vi "Read Data and Memory Array_RageATE.vi"(0 "VISA resource name":refnum<visa-resource-name>, 1 "Channel (1)":i32=1, 3 "Trace":i32=1, 5 "Source (0: Data)":u16(ring) items=["Data", "Memory"], 9 "Correction (0: Data)":u16(ring) items=["Formatted", "Corrected"], 11 "error in (no error)":errorcluster) -> (2 "dB":dbl[](array[numeric]), 4 "VISA resource name out":refnum<visa-resource-name>, 6 "Primary / Real":dbl[](array[numeric]), 10 "Secondary / Imaginary":dbl[](array[numeric]), 15 "error out":errorcluster)   [LabVIEW 2018, in "Agilent ENA Series.lvlib"]
doc: "Reads out the formated or corrected data or memory array, for the active trace of selected channel."
uses:
  Agilent ENA Series.lvlib
panel:
  out "size(s) 2":i32
  out "size(s)":i32
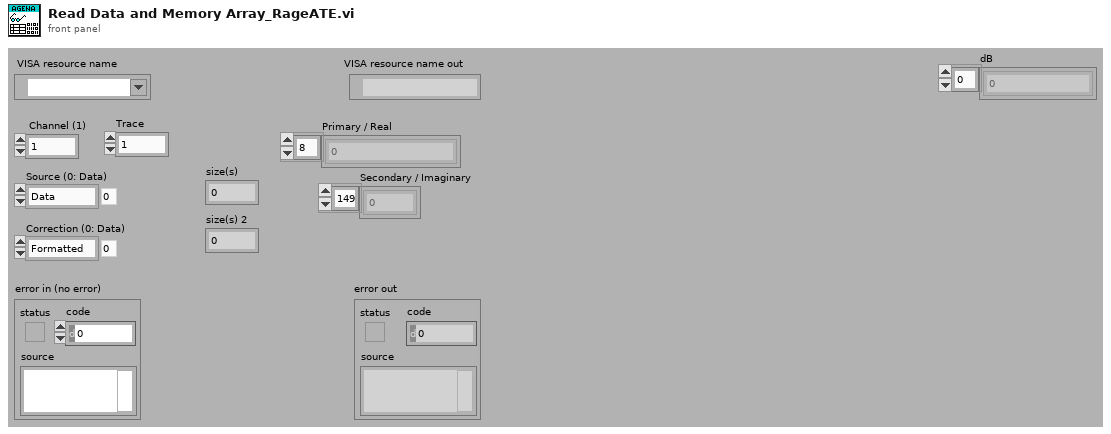
[diagram p1: front panel]
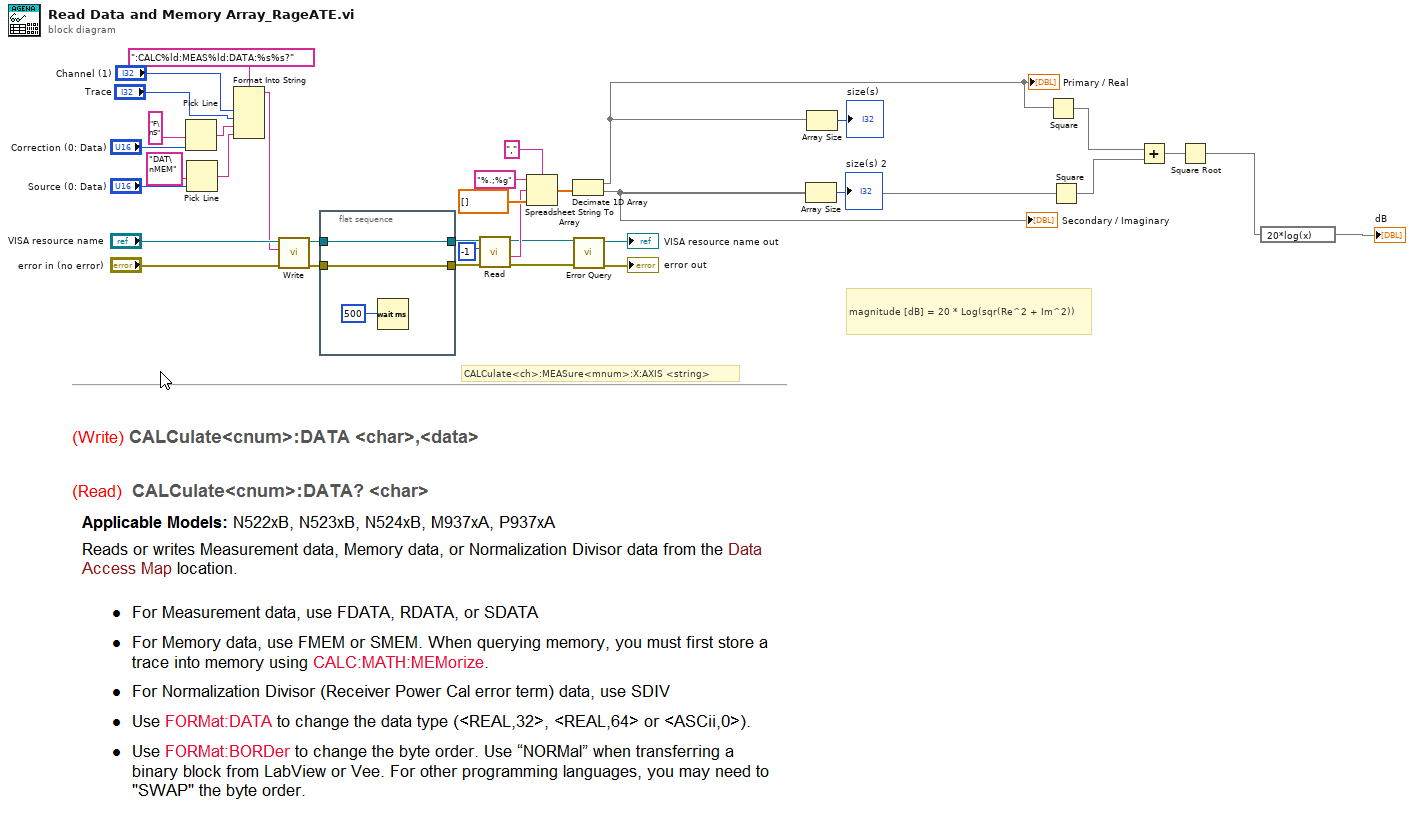
[diagram p0: block diagram]
diagram:
  # "magnitude [dB] = 20 * Log(sqr(Re^2 + Im^2))"
  # "CALCulate<ch>:MEASure<mnum>:X:AXIS <string>"
  n1 = Pick Line(multi-line string="F\nS", line index="Correction (0: Data)") -> (output string=w25:string)  [unwired: 1 in]
  n2 = Pick Line(multi-line string="DAT\nMEM", line index="Source (0: Data)") -> (output string=w22:string)  [unwired: 1 in]
  n3 = Format Into String(format string=":CALC%ld:MEAS%ld:DATA:%s%s?", "Channel (1)", "Trace", w25, w22) -> (resulting string=w31:string)  [unwired: 2 in, 1 out]
  n4 = call "Write.vi"("error in (no error)"="error in (no error)", "String ()"=w31, "VISA resource name"="VISA resource name") -> ("error out"=w16:errorcluster, "VISA resource name out"=w18:refnum<visa-resource-name>)  [unwired: 6 in, 1 out]
  n5 = flat-sequence {
    tunnel: w18 -> [w38]
    tunnel: [w38] -> w17
    tunnel: w16 -> [w37]
    tunnel: [w37] -> w15
    frame #0 {
      n6 = Wait (ms)(milliseconds to wait=u32 500) -> ()  [unwired: 1 out]
    }
  }
  n7 = call "Read.vi"("error in (no error)"=w15, "Number Of Bytes"=-1, "VISA resource name"=w17) -> ("error out"=w13:errorcluster, "String"=w21:string, "VISA resource name out"=w14:refnum<visa-resource-name>)  [unwired: 5 in, 1 out]
  n8 = Spreadsheet String To Array(delimiter (Tab)=",", format string="%.;%g", spreadsheet string=w21, array type (2D Dbl)=dbl[] []) -> (array=w19:dbl[])
  n9 = Decimate 1D Array(w19) -> (w7:dbl[], w6:dbl[])
  "Primary / Real" <- w7
  "Secondary / Imaginary" <- w6
  n10 = call "Error Query.vi"("error in (no error)"=w13, "VISA resource name"=w14) -> ("error out"=→"error out":errorcluster, "VISA resource name out"=→"VISA resource name out":refnum<visa-resource-name>)  [unwired: 6 in, 2 out]
  n11 = Array Size(array=w6) -> (size(s)=→"size(s) 2":i32)
  n12 = Array Size(array=w7) -> (size(s)=→"size(s)":i32)
  n13 = Square(x=w7) -> (x^2=w5:dbl[])
  n14 = Square(x=w6) -> (x^2=w4:dbl[])
  n15 = Add(x=w5, y=w4) -> (x+y=w3:dbl[])
  n16 = Square Root(x=w3) -> (sqrt(x)=w2:dbl[])
  n17 = expression code="20*log(x)"(w2) -> (→"dB":dbl[])
